vi "07Foot.vi"() -> ()   [LabVIEW 2020]
uses:
  <resource>/objmgr/daqmx.rc
  <vilib>/DAQmx/configure/timing.llb/DAQmx Timing (Sample Clock).vi
  <vilib>/Utility/file.llb/Read Delimited Spreadsheet (DBL).vi
  <vilib>/DAQmx/create/channels.llb/DAQmx Create Channel (DI-Digital Input).vi
  <vilib>/Utility/file.llb/Write Delimited Spreadsheet (DBL).vi
  <vilib>/Instr/_visa.llb/VISA Configure Serial Port (Serial Instr).vi
  07FootGlobals.vi
panel:
  in  "Tab Control":enum32{"Page 1", "Page 2"}(tab)
  out "NEXT DURATION":dbl format="%#.1f"
  out "NEXT MPH":dbl min=0.0 max=12.0 step=0.1 format="%.1f"
  out "Time Left":dbl format="%#.0f"
  out "ESTOP":bool
  in  "ESTOP RESUME":bool
  out "MPH":dbl min=0.0 max=12.0 step=0.1 format="%.1f"
  out "ESTOP2":bool
  out "Report Location":path
  in  "TestScript":path=path "C:/LabVIEW VIs/TRMConsole/FootTime.txt"
  out "Waveform Graph":dbl[](graph)
  out "speed":dbl[](array[numeric])
  out "time":dbl[](array[numeric])
  out "dwell":dbl[](array[numeric])
  out "step":i32
  out "arraysize":i32
  out "x-y":u32
  out "appended path":path
  out "stopping":bool
  out "String":string
  in  "stop":bool
  out "MPH READ":u8
  in  "Serial Port":refnum<visa-resource-name>="COM8"
  in  "lines":tag="DAQMod1/port0"
  out "Enum":T1(ring)
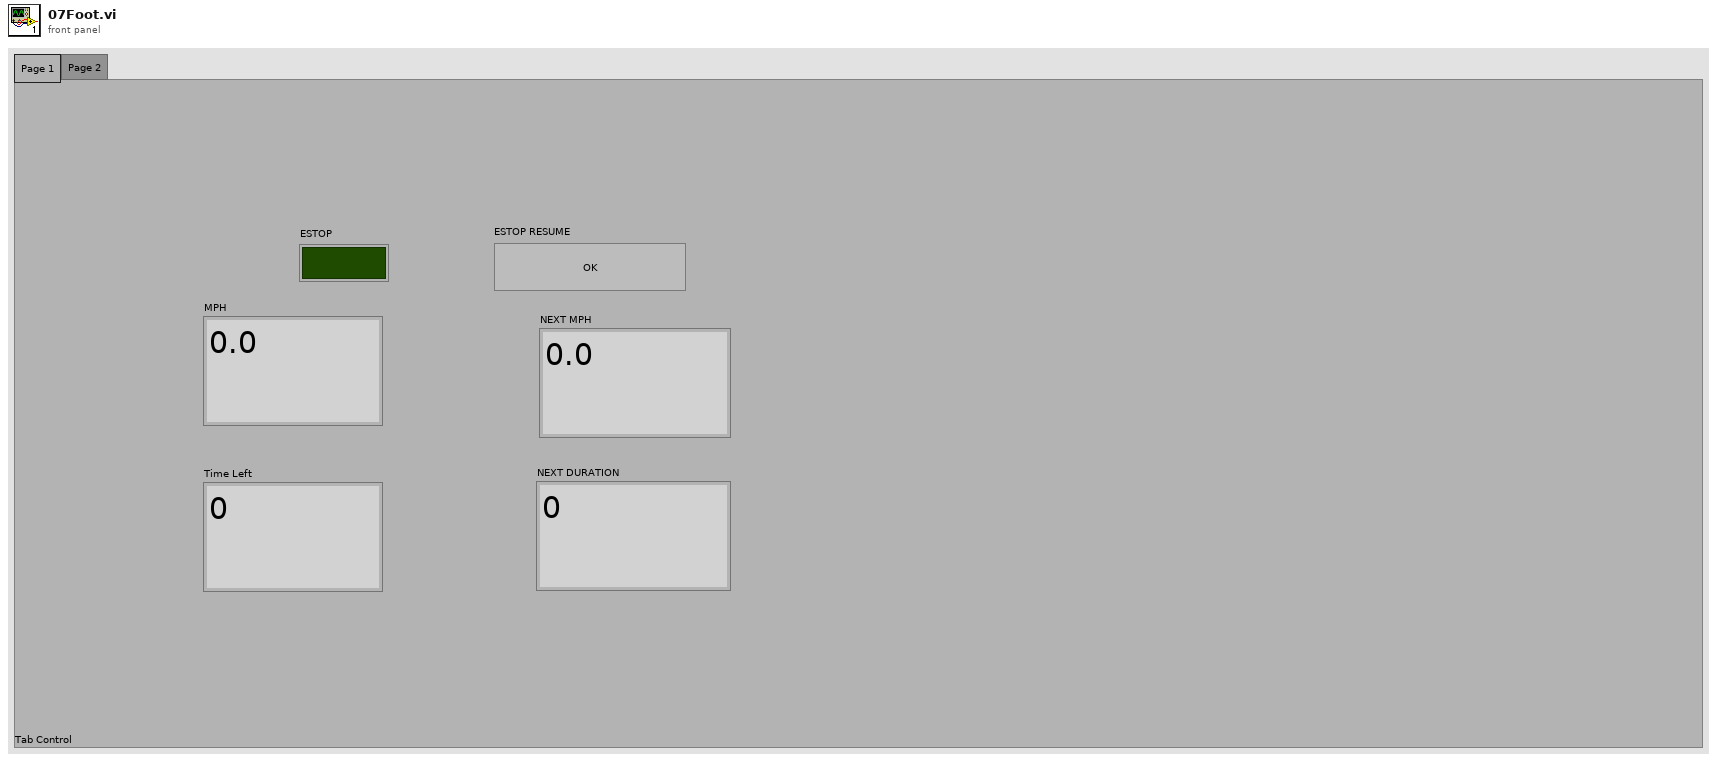
[diagram p1: front panel]
types:
  T1 = enum16{"Initialize", "SetMPH", "GetData", "CheckTiming", "CompressWave", "StartDAQ", "StopDAQ", "Dwell", "WaitforMPH", "ESTOP Wait", "ESTOP Resume"}
  T2 = enum16{"Initialize", "SetMPH", "GetData", "CheckTiming", "CompressWave", "StartDAQ", "StopDAQ", "Dwell", "WaitforMPH"}
  T3 = enum16{"Initialize", "SetMPH", "GetData", "CheckTiming", "CompressWave", "StartDAQ"}
  T4 = enum16{"Initialize", "SetMPH", "GetData", "CheckTiming", "CompressWave"}
  T5 = enum16{"Initialize", "SetMPH", "GetData", "CheckTiming", "CompressWave", "StartDAQ", "StopDAQ"}
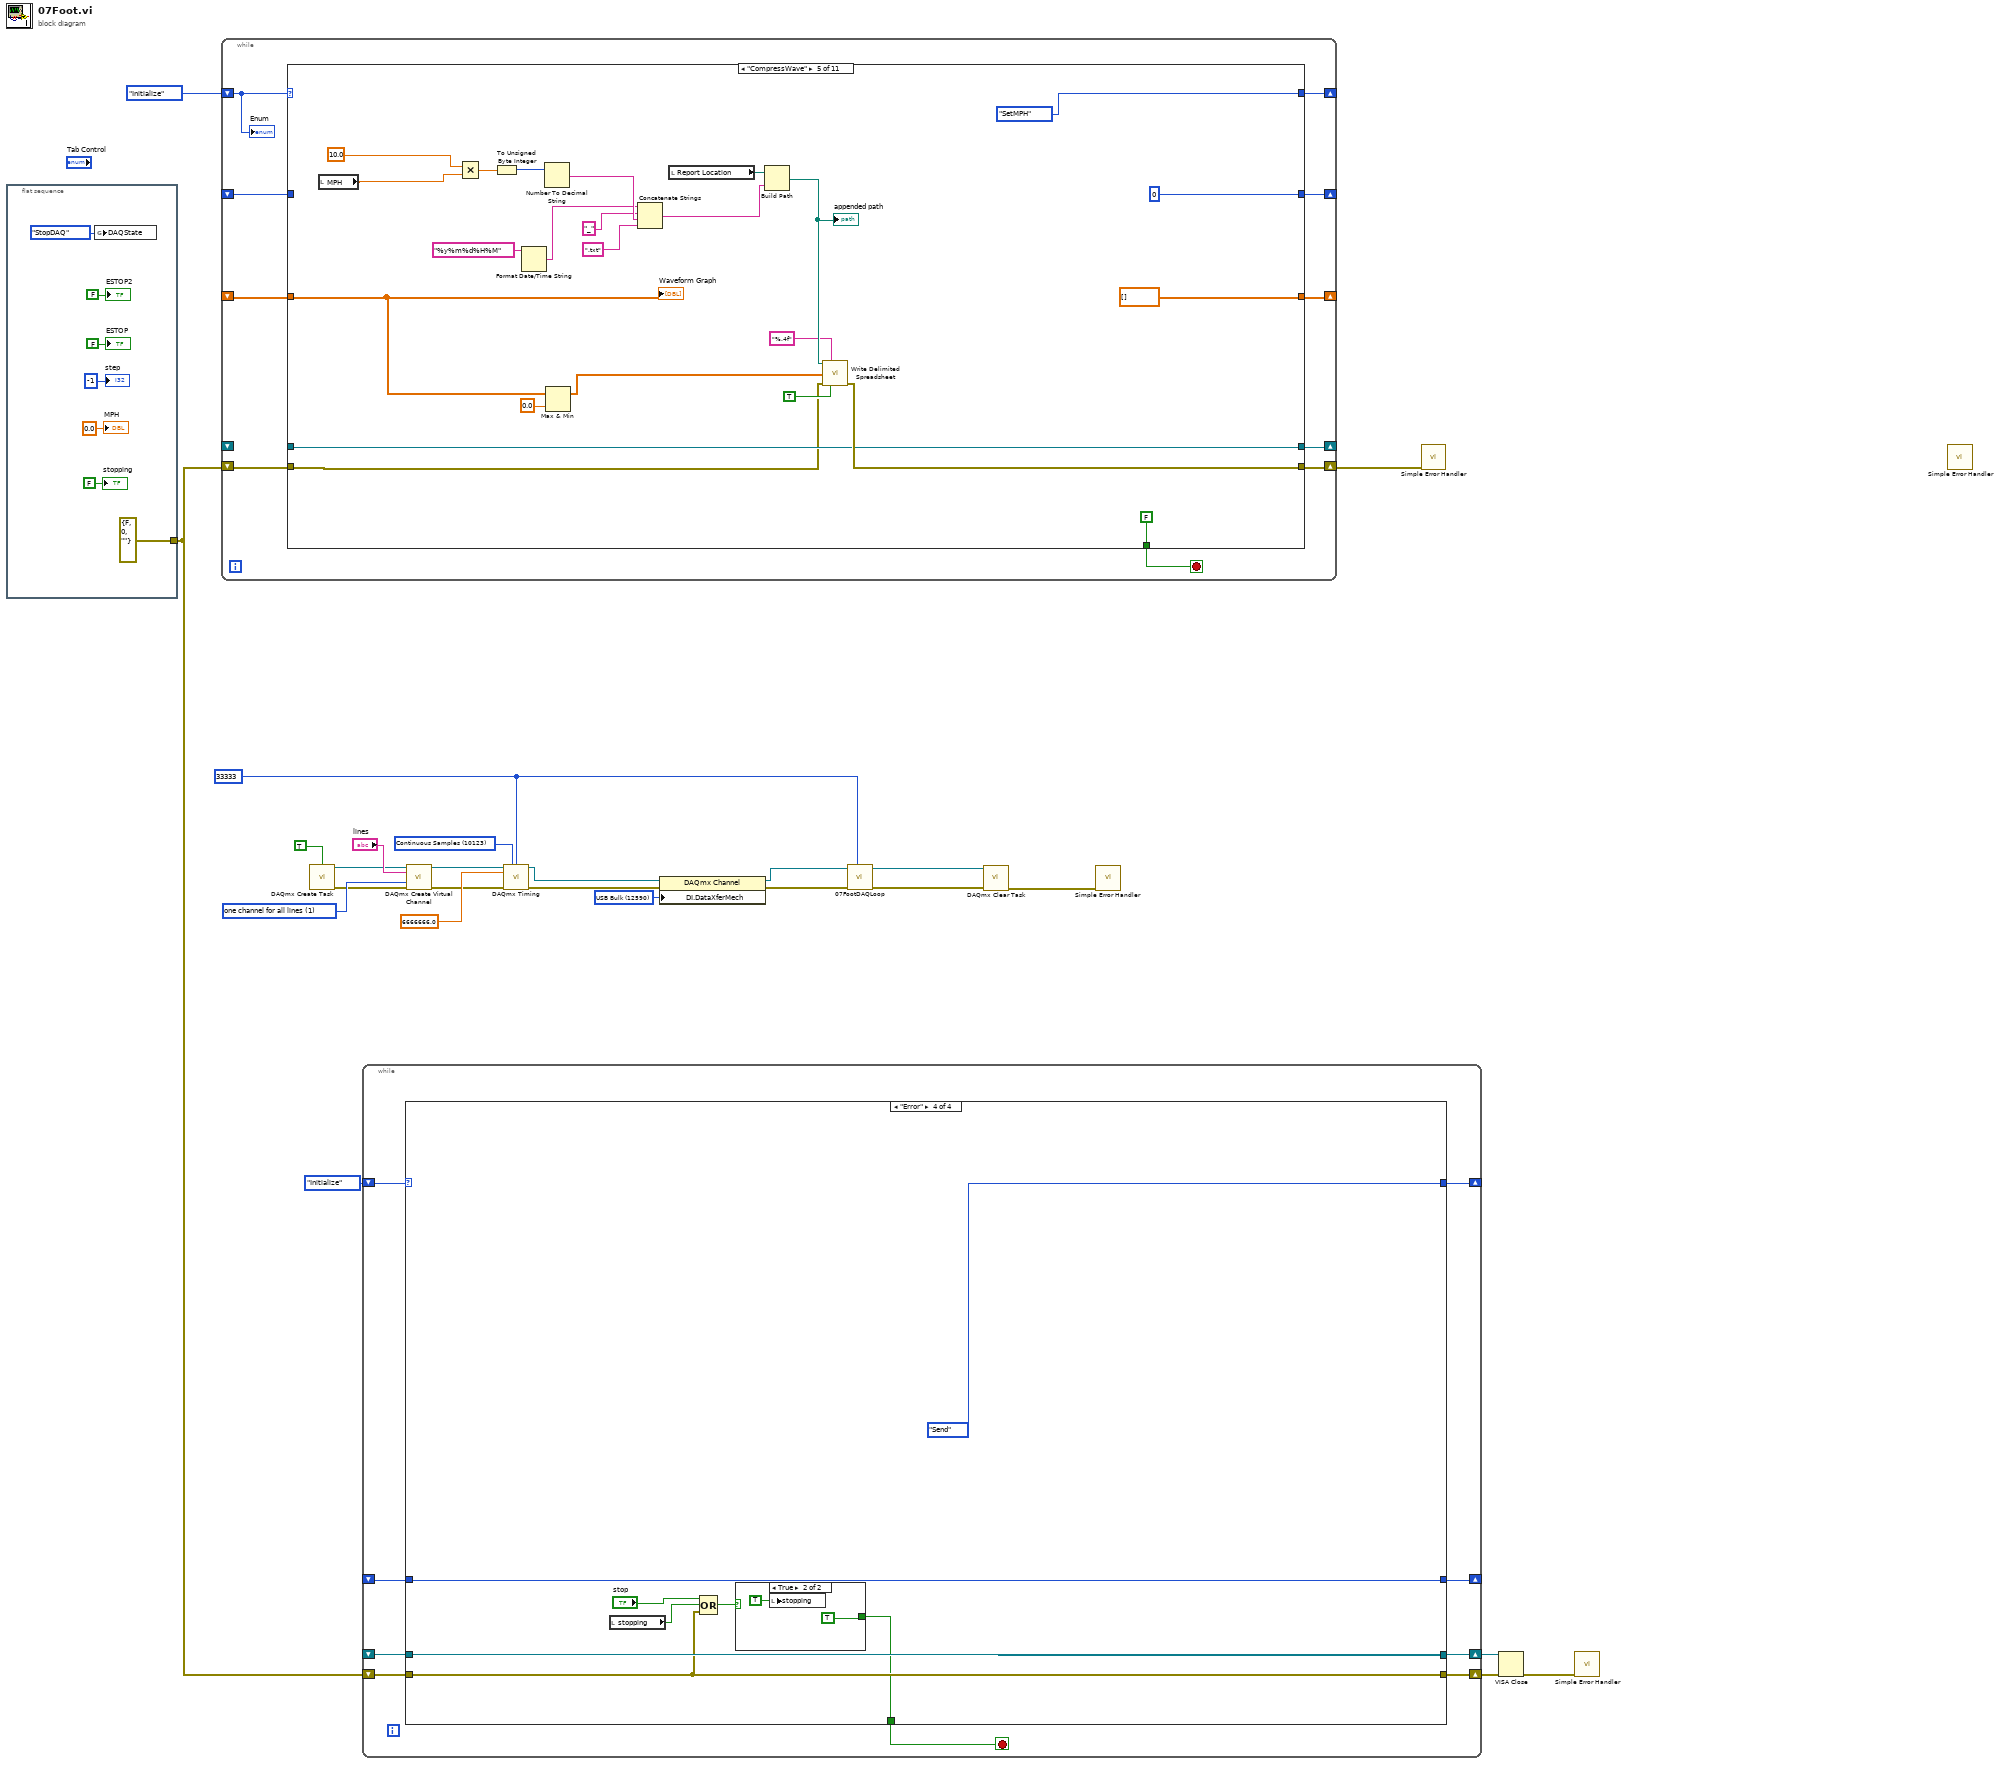
[diagram p0: block diagram]
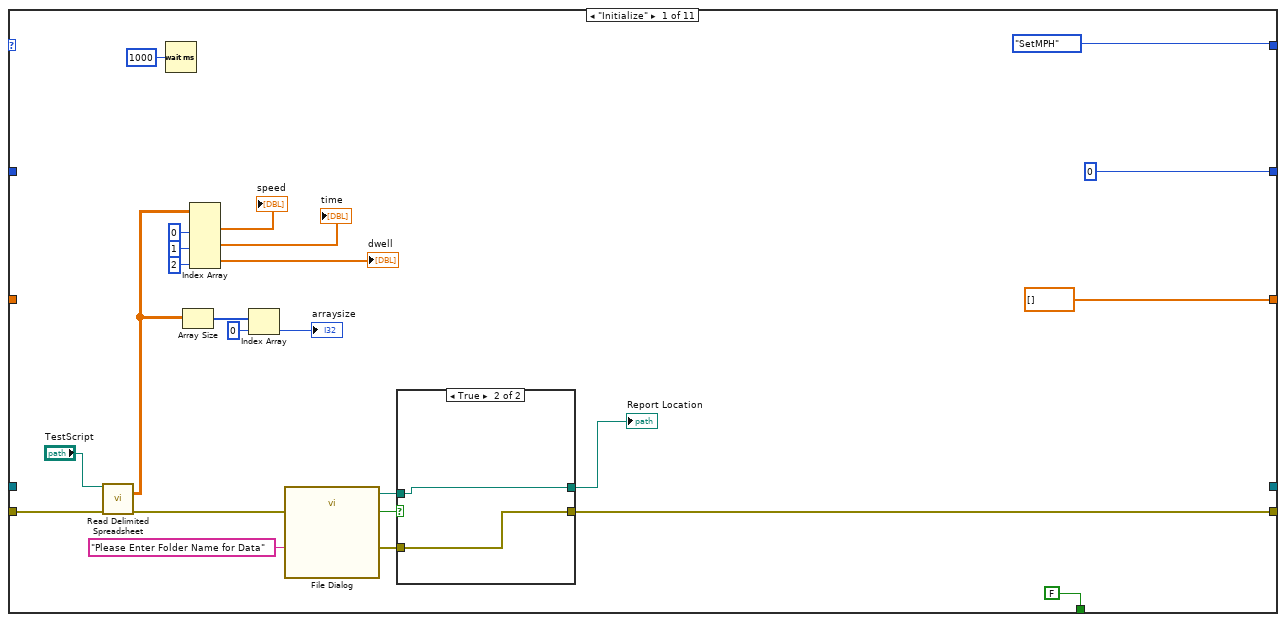
[diagram p2: hidden frame]
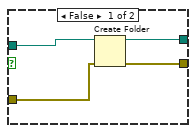
[diagram p3: hidden frame]
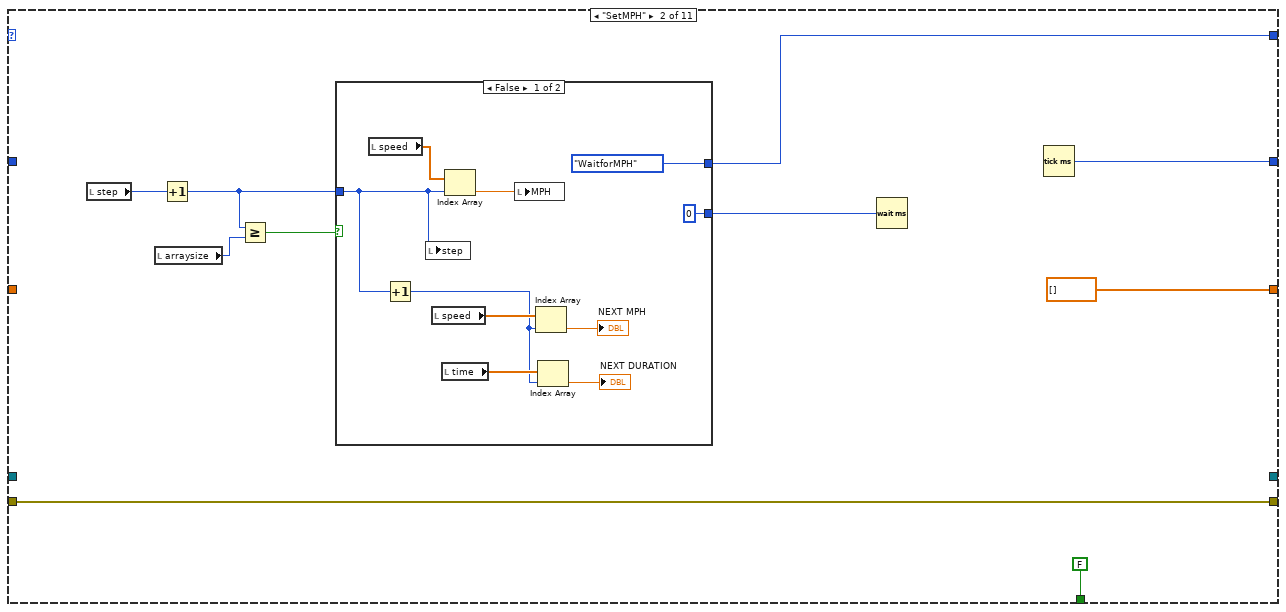
[diagram p4: hidden frame]
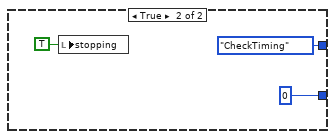
[diagram p5: hidden frame]
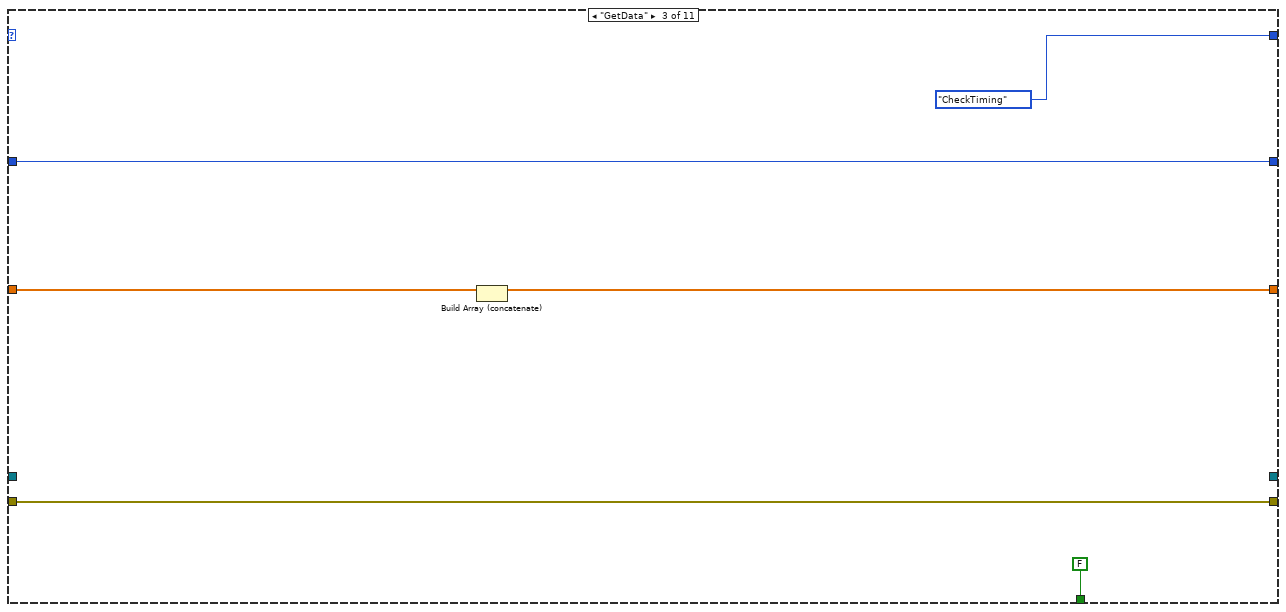
[diagram p6: hidden frame]
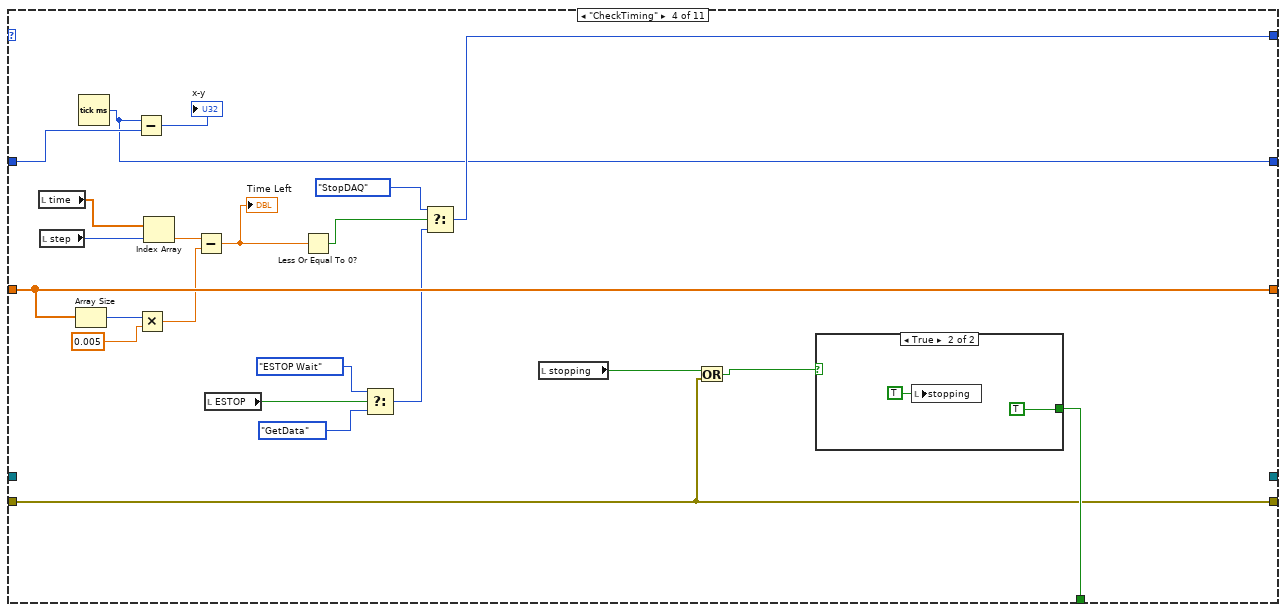
[diagram p7: hidden frame]
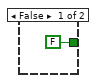
[diagram p8: hidden frame]
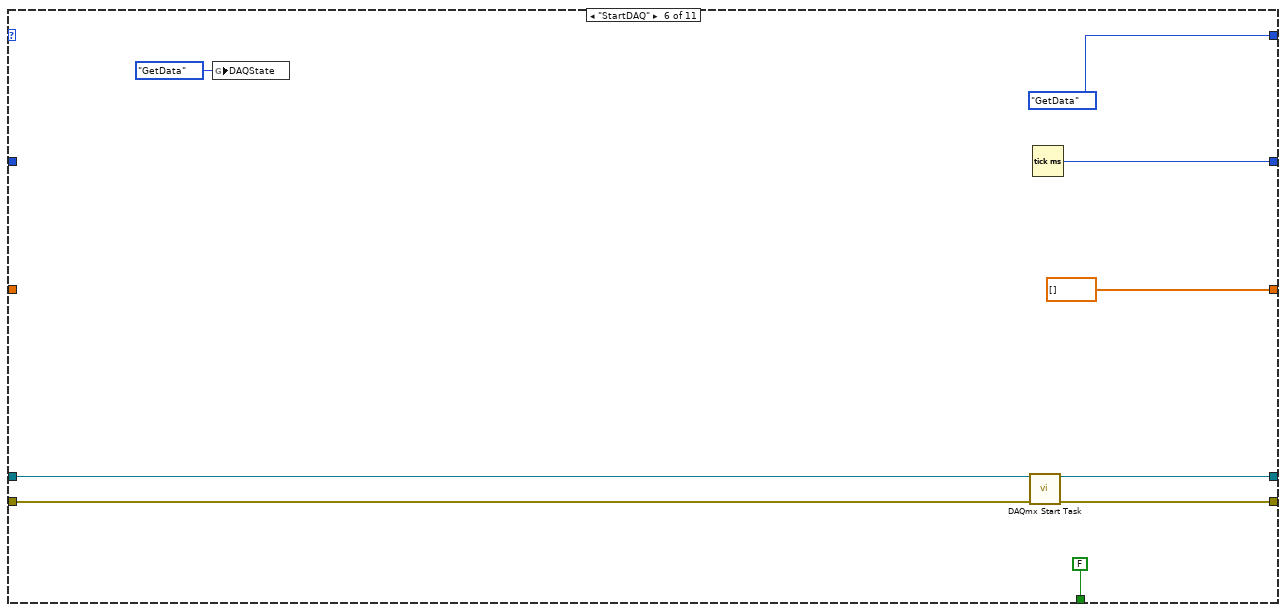
[diagram p9: hidden frame]
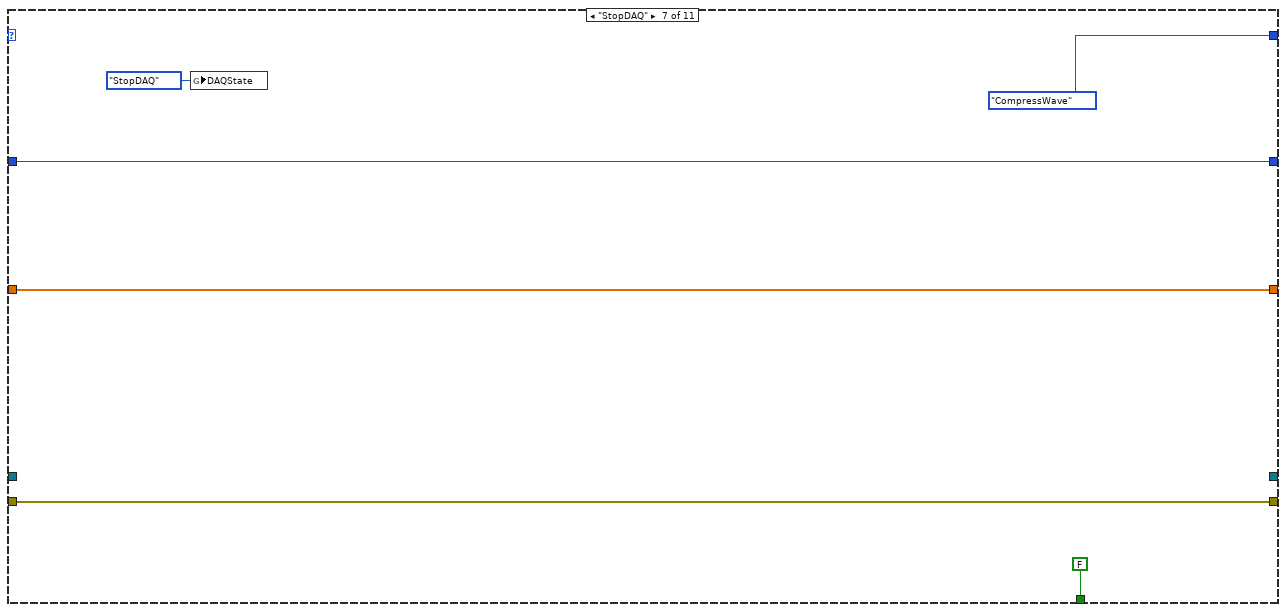
[diagram p10: hidden frame]
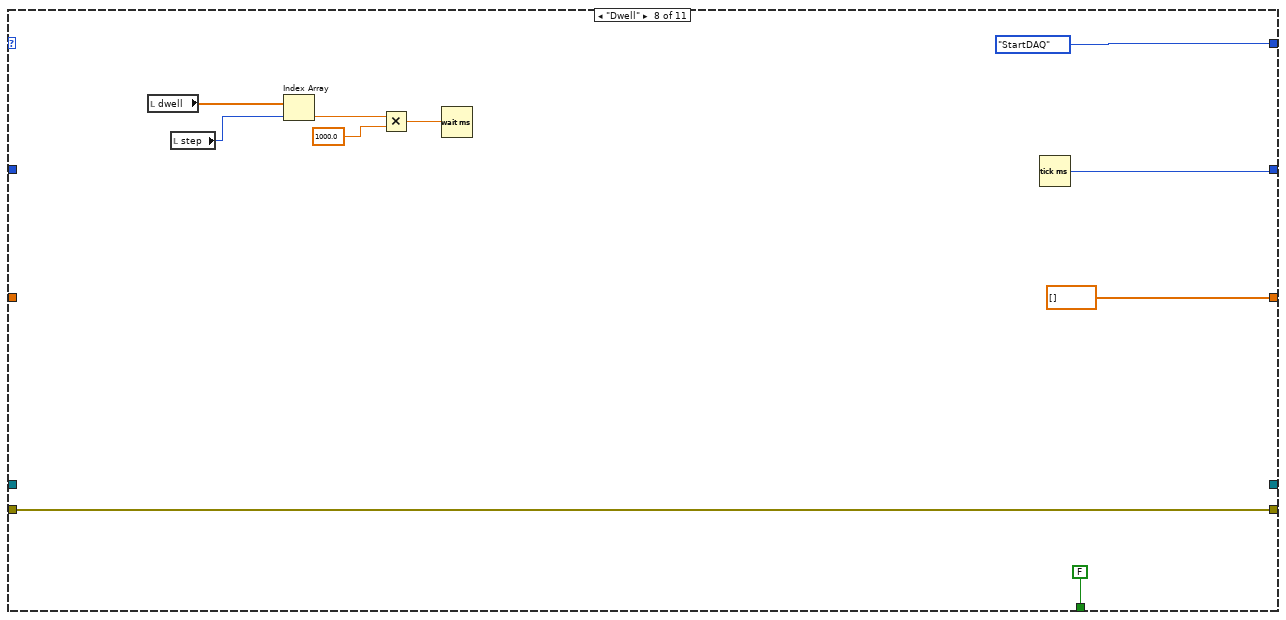
[diagram p11: hidden frame]
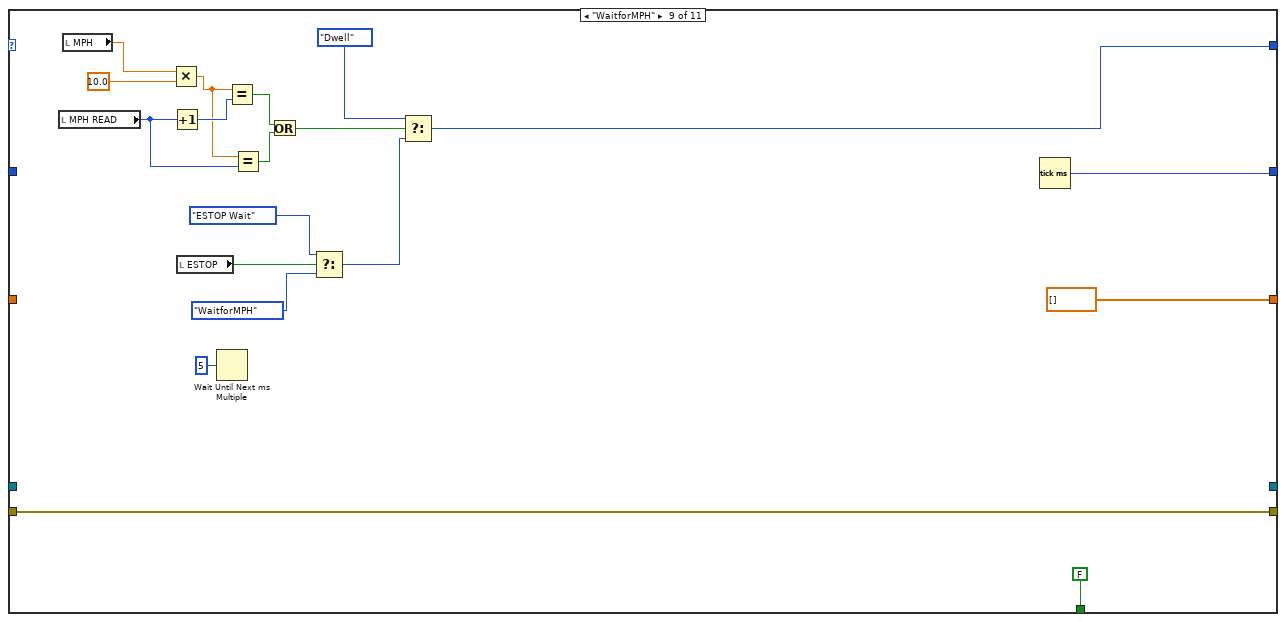
[diagram p12: hidden frame]
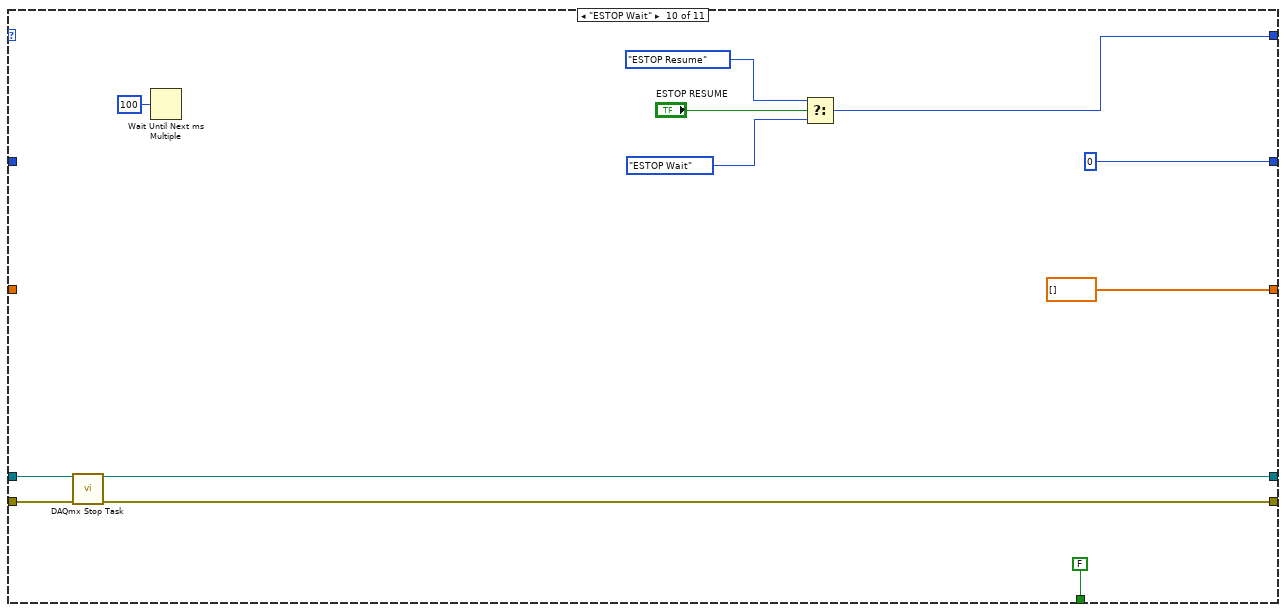
[diagram p13: hidden frame]
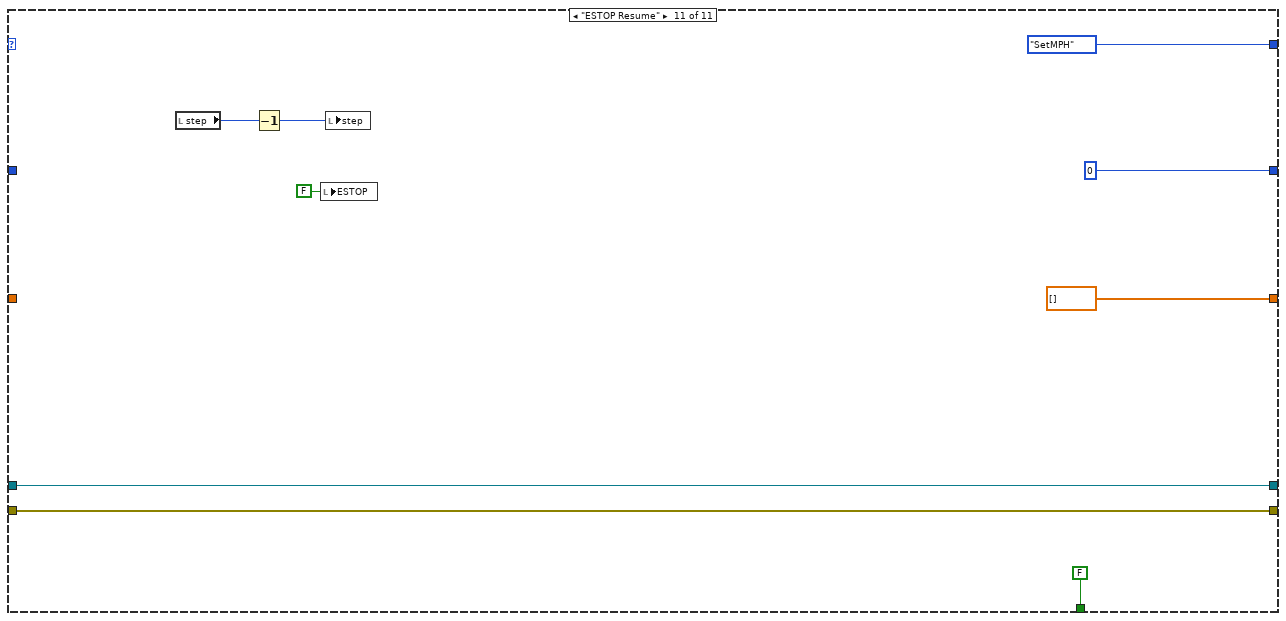
[diagram p14: hidden frame]
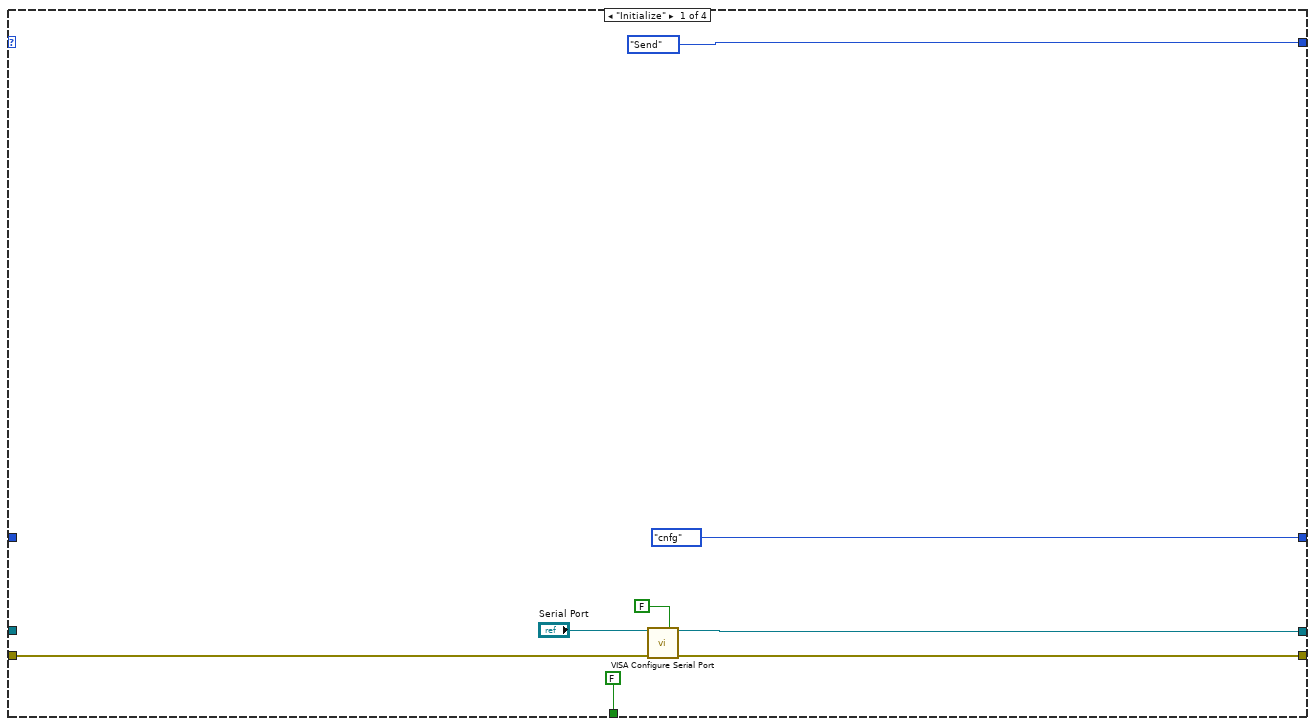
[diagram p15: hidden frame]
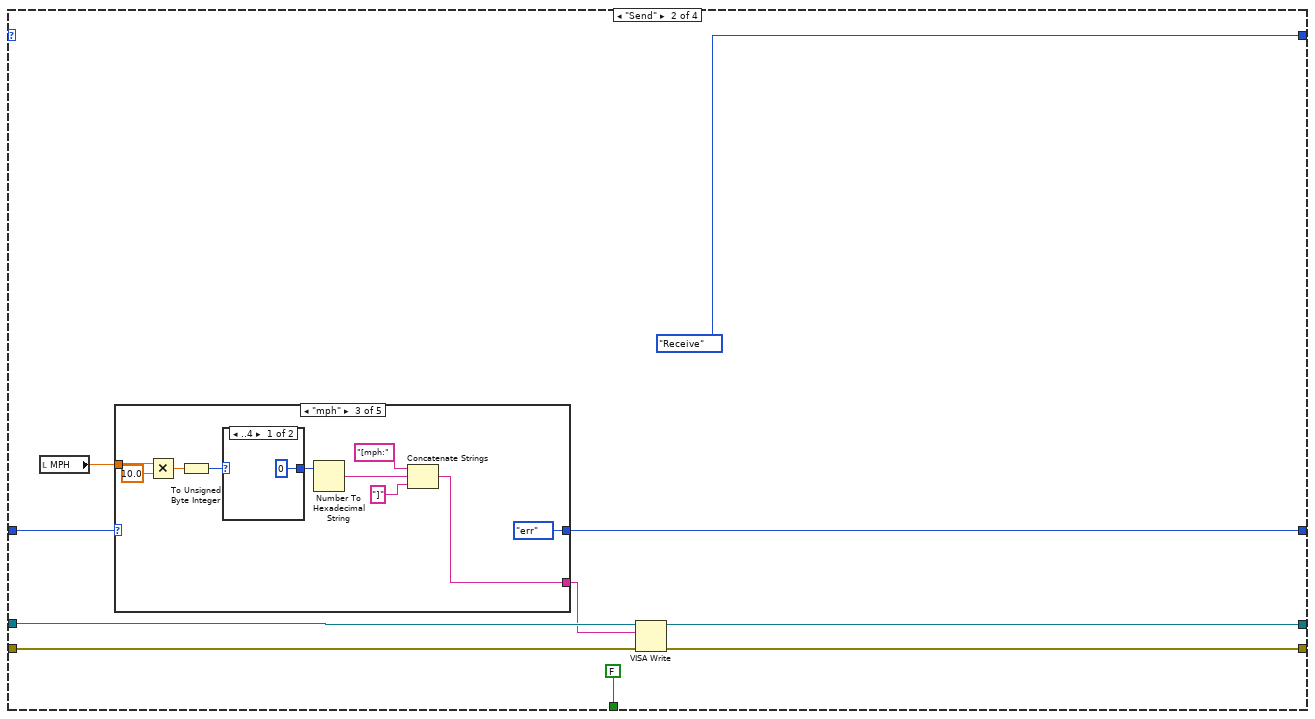
[diagram p16: hidden frame]
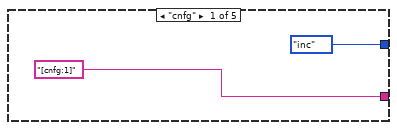
[diagram p17: hidden frame]
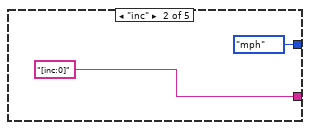
[diagram p18: hidden frame]
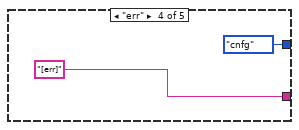
[diagram p20: hidden frame]
diagram:
  w19 = 12590 items=["DMA"=10054, "Interrupts"=10204, "Programmed I/O"=10264, "USB Bulk"=12590] ("DI.DataXferMech")
  w15 = 10123 items=["Finite Samples"=10178, "Continuous Samples"=10123, "Hardware Timed Single Point"=12522] ("sample mode")
  w10 = 1 items=["one channel for each line", "one channel for all lines"] ("line grouping")
  w5 = 33333 ("samples per channel")
  n1 = flat-sequence {
    tunnel: [errorcluster {"status"=FALSE, "code"=0, "source"=""} ("error constant")] -> w20
    frame #0 {
      n2 = global write "07FootGlobals.vi" "DAQState"(enum16{"GetData", "StopDAQ"}."StopDAQ" ("DAQState")) -> ()
      "stopping" <- FALSE ("stopping")
      "MPH" <- 0.0 ("MPH")
      "step" <- -1 ("step")
      "ESTOP" <- FALSE ("ESTOP")
      "ESTOP2" <- FALSE ("ESTOP2")
    }
  }
  n3 = while {
    shift-right: [w42] -> _
    shift-left: T1."Initialize" -> [w33]
    shift-right: [w40] -> _
    shift-left: _ -> [_]
    shift-right: [w39] -> w1
    shift-left: w20 -> [w38]
    shift-right: [w37] -> _
    shift-left: _ -> [w36]
    shift-right: [w35] -> _
    shift-left: _ -> [w34]
    stop <- w41 stop-if-true
    n4 = case shown="\"CompressWave\"" w33 {
      tunnel: [T1."SetMPH" w77 T4."CheckTiming" w117 T1."SetMPH" T3."GetData" T5."CompressWave" T2."StartDAQ" w187 w201 T1."SetMPH" ("f")] -> w42
      tunnel: [FALSE FALSE FALSE w122 FALSE FALSE FALSE FALSE FALSE FALSE FALSE] -> w41
      tunnel: [_ _ _ _ w134 w154 _ _ _ w196 w209] -> w40
      tunnel: [w43 w79 w96 w118 w147 w155 w161 w173 w192 w195 w210] -> w39
      tunnel: _ -> [_ _ _ _ w134 w153 _ _ _ w198 w209]
      tunnel: w38 -> [w62 w79 w96 w118 w133 w152 w161 w173 w192 w197 w210]
      tunnel: [u32 0 w78 w100 w102 u32 0 w158 w162 w175 w194 u32 0 ("millisecond timer value") u32 0 ("millisecond timer value")] -> w37
      tunnel: w36 -> [_ _ w100 w121 _ _ w162 _ _ _ _]
      tunnel: [dbl[] [] dbl[] [] w99 w116 dbl[] [] dbl[] [] w164 dbl[] [] dbl[] [] dbl[] [] dbl[] []] -> w35
      tunnel: w34 -> [_ _ w98 w116 w128 _ w164 _ _ _ _]
      frame "Initialize" {
        n5 = call-poly <vilib>:"Read Delimited Spreadsheet.vi"("file path (dialog if empty)"="TestScript", "error in (no error)"=w62) -> ("all rows"=w52:dbl[][], "error out"=w50:errorcluster)  [unwired: 8 in, 4 out]
        n6 = Wait (ms)(milliseconds to wait=u32 1000) -> ()  [unwired: 1 out]
        n7 = Array Size(array=w52) -> (size(s)=w55:i32[])
        n8 = Index Array(array=w52, index (col) #1=0 ("disabled index (col)"), index (col) #2=1 ("index (col)"), index (col) #3=2 ("index (col)")) -> (element #1=→"speed":dbl[], element #2=→"time":dbl[], element #3=→"dwell":dbl[])  [unwired: 3 in]
        n9 = Index Array(array=w55, index=0) -> (element=→"arraysize":i32)
        n10 = call "File Dialog"("prompt"="Please Enter Folder Name for Data", "error in"=w50) -> ("selected path"=w46:path, "exists"=w48:bool, "error out"=w47:errorcluster)  [unwired: 10 in, 1 out]
        n11 = case shown="True" w48 {
          tunnel: w47 -> [w70 w71]
          tunnel: w46 -> [w69 w72]
          tunnel: [w68 w71] -> w43
          tunnel: [w67 w72] -> w45
          frame False {
            n12 = Create Folder(path (use dialog)=w69, error in=w70) -> (created path=w67:path, error out=w68:errorcluster)  [unwired: 1 in, 1 out]
          }
          frame True {
          }
        }
        "Report Location" <- w45
      }
      frame "SetMPH" {
        n13 = local read "step"() -> (w74:i32)
        n14 = local read "arraysize"() -> (w76:i32)
        n15 = Increment(x=w74) -> (x+1=w73:i32)
        n16 = Greater Or Equal?(x=w73, y=w76) -> (x >= y?=w75:bool)
        n17 = case shown="False" w75 {
          tunnel: [u32 0 ("milliseconds to wait") u32 0 ("milliseconds to wait")] -> w81
          tunnel: [T2."WaitforMPH" T3."CheckTiming"] -> w77
          tunnel: w73 -> [w88 _]
          frame False {
            n18 = local read "speed"() -> (w91:dbl[])
            n19 = Increment(x=w88) -> (x+1=w83:i32)
            n20 = local write "step"(w88) -> ()
            n21 = local read "speed"() -> (w87:dbl[])
            n22 = local read "time"() -> (w84:dbl[])
            n23 = Index Array(array=w91, index=w88) -> (element=w90:dbl)
            n24 = local write "MPH"(w90) -> ()
            n25 = Index Array(array=w87, index=w83) -> (element=→"NEXT MPH":dbl)
            n26 = Index Array(array=w84, index=w83) -> (element=→"NEXT DURATION":dbl)
          }
          frame True {
            n27 = local write "stopping"(TRUE ("stopping")) -> ()
          }
        }
        n28 = Wait (ms)(milliseconds to wait=w81) -> ()  [unwired: 1 out]
        n29 = Tick Count (ms)() -> (millisecond timer value=w78:u32)
      }
      frame "GetData" {
        n30 = Build Array (concatenate)(w98) -> (w99:dbl[])  [unwired: 1 in]
      }
      frame "CheckTiming" {
        n31 = local read "time"() -> (w113:dbl[])
        n32 = local read "step"() -> (w112:i32)
        n33 = Array Size(array=w116) -> (size(s)=w115:i32)
        n34 = Tick Count (ms)() -> (millisecond timer value=w102:u32)
        n35 = Subtract(x=w102, y=w121) -> (x-y=→"x-y":u32)
        n36 = Multiply(x=w115, y=0.005) -> (x*y=w105:dbl)
        n37 = Index Array(array=w113, index=w112) -> (element=w106:dbl)
        n38 = Subtract(x=w106, y=w105) -> (x-y=w104:dbl)
        "Time Left" <- w104
        n39 = local read "ESTOP"() -> (w109:bool)
        n40 = Less Or Equal To 0?(x=w104) -> (x <= 0?=w103:bool)
        n41 = Select(t=T1."ESTOP Wait", s=w109, f=T1."GetData") -> (s? t:f=w107:T1)
        n42 = Select(t=T1."StopDAQ", s=w103, f=w107) -> (s? t:f=w117:T1)
        n43 = local read "stopping"() -> (w120:bool)
        n44 = Or(x=w120, y=w118) -> (x .or. y?=w119:bool)
        n45 = case shown="True" w119 {
          tunnel: [FALSE TRUE] -> w122
          frame False {
          }
          frame True {
            n46 = local write "stopping"(TRUE ("stopping")) -> ()
          }
        }
      }
      frame "CompressWave" {
        n47 = local read "MPH"() -> (w137:dbl)
        n48 = Multiply(x=10.0, y=w137) -> (x*y=w140:dbl)
        n49 = To Unsigned Byte Integer(number=w140) -> (unsigned 8bit integer=w139:u8)
        n50 = Format Date/Time String(time format string (%c)="%y%m%d%H%M") -> (date/time string=w129:string)  [unwired: 2 in]
        n51 = Number To Decimal String(number=w139) -> (decimal integer string=w138:string)  [unwired: 1 in]
        n52 = Max & Min(x=w128, y=0.0) -> (max(x,y)=w135:dbl[])  [unwired: 1 out]
        n53 = Concatenate Strings(w129, "_" ("string"), w138, ".txt" ("string")) -> (w143:string)
        n54 = local read "Report Location"() -> (w132:path)
        n55 = Build Path(base path=w132, name or relative path=w143) -> (appended path=w142:path)
        "appended path" <- w142
        n56 = call-poly <vilib>:"Write Delimited Spreadsheet.vi"("file path (dialog if empty)"=w142, "format (%.3f)"="%.4f", "1D data"=w135, "error in (no error)"=w133, "transpose? (no:F)"=TRUE ("transpose? (F)")) -> ("error out"=w147:errorcluster)  [unwired: 9 in, 1 out]
        "Waveform Graph" <- w128
      }
      frame "StartDAQ" {
        n57 = global write "07FootGlobals.vi" "DAQState"(enum16{"GetData", "StopDAQ", "Quit"}."GetData" ("DAQState")) -> ()
        n58 = call <vilib>:"DAQmx Start Task.vi"("task/channels in"=w153, "error in"=w152) -> ("task out"=w154:refnum<k21>, "error out"=w155:errorcluster)  [unwired: 12 in]
        n59 = Tick Count (ms)() -> (millisecond timer value=w158:u32)
      }
      frame "StopDAQ" {
        n60 = global write "07FootGlobals.vi" "DAQState"(enum16{"GetData", "StopDAQ", "Quit"}."StopDAQ" ("DAQState")) -> ()
      }
      frame "Dwell" {
        n61 = local read "dwell"() -> (w171:dbl[])
        n62 = local read "step"() -> (w170:i32)
        n63 = Index Array(array=w171, index=w170) -> (element=w169:dbl)
        n64 = Multiply(x=w169, y=1000.0) -> (x*y=w167:dbl)
        n65 = Wait (ms)(milliseconds to wait=w167) -> ()  [unwired: 1 out]
        n66 = Tick Count (ms)() -> (millisecond timer value=w175:u32)
      }
      frame "WaitforMPH" {
        n67 = local read "MPH READ"() -> (w179:u8)
        n68 = local read "MPH"() -> (w190:dbl)
        n69 = Multiply(x=w190, y=10.0) -> (x*y=w180:dbl)
        n70 = Increment(x=w179) -> (x+1=w188:u8)
        n71 = local read "ESTOP"() -> (w185:bool)
        n72 = Wait Until Next ms Multiple(millisecond multiple=u32 5) -> ()  [unwired: 1 out]
        n73 = Equal?(x=w180, y=w188) -> (x = y?=w177:bool)
        n74 = Equal?(x=w180, y=w179) -> (x = y?=w178:bool)
        n75 = Or(x=w177, y=w178) -> (x .or. y?=w176:bool)
        n76 = Select(t=T1."ESTOP Wait", s=w185, f=T1."WaitforMPH") -> (s? t:f=w182:T1)
        n77 = Select(t=T1."Dwell", s=w176, f=w182) -> (s? t:f=w187:T1)
        n78 = Tick Count (ms)() -> (millisecond timer value=w194:u32)
      }
      frame "ESTOP Wait" {
        n79 = call <vilib>:"DAQmx Stop Task.vi"("task/channels in"=w198, "error in"=w197) -> ("task out"=w196:refnum<k21>, "error out"=w195:errorcluster)  [unwired: 12 in]
        n80 = Wait Until Next ms Multiple(millisecond multiple=u32 100) -> ()  [unwired: 1 out]
        n81 = Select(t=T1."ESTOP Resume", s="ESTOP RESUME", f=T1."ESTOP Wait") -> (s? t:f=w201:T1)
      }
      frame "ESTOP Resume" {
        n82 = local read "step"() -> (w215:i32)
        n83 = Decrement(x=w215) -> (x-1=w214:i32)
        n84 = local write "ESTOP"(FALSE ("ESTOP")) -> ()
        n85 = local write "step"(w214) -> ()
      }
    }
    "Enum" <- w33
  }
  n86 = call <vilib>:"DAQmx Create Task.vi"("auto cleanup"=TRUE) -> ("task out"=w8:refnum<k21>, "error out"=w9:errorcluster)  [unwired: 13 in]
  n87 = while {
    shift-right: [w220] -> w23
    shift-left: w20 -> [w224]
    shift-right: [w221] -> w24
    shift-left: _ -> [w223]
    shift-right: [w219] -> _
    shift-left: enum16{"Initialize", "Send", "Receive", "Error"}."Initialize" -> [w222]
    shift-right: [w218] -> _
    shift-left: _ -> [w217]
    stop <- w216 stop-if-true
    n88 = case shown="\"Error\"" w222 {
      tunnel: w224 -> [w228 w240 w279 w299]
      tunnel: w223 -> [_ w239 w278 w303]
      tunnel: [w230 w242 w277 w303] -> w221
      tunnel: [w229 w241 w271 w299] -> w220
      tunnel: [enum16{"Initialize", "Send", "Receive", "Error"}."Send" enum16{"Initialize", "Send", "Receive", "Error"}."Receive" enum16{"Initialize", "Send", "Receive", "Error"}."Error" enum16{"Initialize", "Send", "Receive", "Error"}."Send"] -> w219
      tunnel: [enum16{"cnfg", "inc", "mph", "err", "RSET"}."cnfg" w236 w265 w304] -> w218
      tunnel: w217 -> [_ w237 w272 w304]
      tunnel: [FALSE FALSE FALSE w298] -> w216
      frame "Initialize" {
        n89 = call-poly "VISA Configure Serial Port"("VISA resource name"="Serial Port", "Enable Termination\nChar (T)"=FALSE ("Enable Termination\nChar (T)"), "error in (no error)"=w228) -> ("VISA resource name out"=w230:refnum<visa-resource-name>, "error out"=w229:errorcluster)  [unwired: 11 in]
      }
      frame "Send" {
        n90 = local read "MPH"() -> (w233:dbl)
        n91 = case shown="\"mph\"" w237 {
          tunnel: ["[cnfg:1]" "[inc:0]" w247 "[err]" "[RSET]"] -> w238
          tunnel: w233 -> [_ _ w256 _ _]
          tunnel: [enum16{"cnfg", "inc", "mph", "err", "RSET"}."inc" enum16{"cnfg", "inc", "mph", "err", "RSET"}."mph" enum16{"cnfg", "inc", "mph", "err", "RSET"}."err" enum16{"cnfg", "inc", "mph", "err", "RSET"}."cnfg" enum16{"cnfg", "inc", "mph", "err", "RSET"}."cnfg"] -> w236
          frame "cnfg" {
          }
          frame "inc" {
          }
          frame "mph" {
            n92 = Multiply(x=w256, y=10.0) -> (x*y=w250:dbl)
            n93 = To Unsigned Byte Integer(number=w250) -> (unsigned 8bit integer=w249:u8)
            n94 = case shown="..4" w249 {
              selector: w249 -> [_ w258]
              tunnel: [u8 0 w258] -> w248
              frame ..4 {
              }
              frame 5.. {
              }
            }
            n95 = Number To Hexadecimal String(2:w248) -> (0:w253:string)  [unwired: 1 in]
            n96 = Concatenate Strings("[mph:" ("string"), w253, "]" ("string")) -> (w247:string)
          }
          frame "err" {
          }
          frame "RSET" {
          }
        }
        n97 = VISA Write(VISA resource name=w239, write buffer=w238, error in (no error)=w240) -> (VISA resource name out=w242:refnum<visa-resource-name>, error out=w241:errorcluster)  [unwired: 1 out]
      }
      frame "Receive" {
        n98 = flat-sequence {
          tunnel: w278 -> [w296]
          tunnel: [w296] -> w283
          frame #0 {
            n99 = Wait Until Next ms Multiple(millisecond multiple=u32 250) -> ()  [unwired: 1 out]
          }
        }
        n100 = property class="Serial Instr"(reference=w283, error in=w279) -> (reference out=w281:refnum<visa-resource-name>, error out=w282:errorcluster, "Bytes at Port"=w280:u32)
        n101 = VISA Read(VISA resource name=w281, byte count=w280, error in (no error)=w282) -> (VISA resource name out=w277:refnum<visa-resource-name>, read buffer=w266:string, error out=w271:errorcluster)  [unwired: 1 out]
        n102 = Match Pattern(string=w266, regular expression="\\[mph:") -> (after substring=w268:string, offset past match=w269:i32)  [unwired: 1 in, 2 out]
        n103 = Match Pattern(string=w266, regular expression="\\[err:") -> (offset past match=w273:i32)  [unwired: 1 in, 3 out]
        n104 = case shown="Default" w269 {
          tunnel: w268 -> [w290 _]
          frame Default {
            n105 = Hexadecimal String To Number(string=w290, default (0uL)=u8 0 ("default (0 I32)")) -> (number=→"MPH READ":u8)  [unwired: 1 in, 1 out]
          }
          frame -1 {
          }
        }
        n106 = case shown="Default" w273 {
          tunnel: [enum16{"cnfg", "inc", "mph", "err", "RSET"}."RSET" w295] -> w267
          tunnel: w272 -> [_ w295]
          tunnel: w266 -> [w291 _]
          frame Default {
            (unwired) "%y%m%d%H%M" ("time format string (%c)")
            n107 = Format Date/Time String() -> (date/time string=w292:string)  [unwired: 3 in]
            n108 = Concatenate Strings(w292, w291) -> (→"String":string)
          }
          frame -1 {
          }
        }
        n109 = Match Pattern(string=w266, regular expression="\\[ESTOP:BAD\\]") -> (offset past match=w264:i32)  [unwired: 1 in, 3 out]
        n110 = case shown="Default" w264 {
          tunnel: w267 -> [_ w287]
          tunnel: [enum16{"cnfg", "inc", "mph", "err", "RSET"}."RSET" w287] -> w265
          frame Default {
            n111 = local write "ESTOP"(TRUE ("ESTOP")) -> ()
            n112 = local write "MPH"(0.0 ("MPH")) -> ()
          }
          frame -1 {
          }
        }
      }
      frame "Error" {
        n113 = local read "stopping"() -> (w300:bool)
        n114 = Compound Arithmetic op=OR("stop", w300, w299) -> (w302:bool)
        n115 = case shown="True" w302 {
          tunnel: [FALSE TRUE] -> w298
          frame False {
          }
          frame True {
            n116 = local write "stopping"(TRUE ("stopping")) -> ()
          }
        }
      }
    }
  }
  n117 = call-poly <vilib>:"DAQmx Create Virtual Channel.vi"("task in"=w8, "lines"="lines", "line grouping"=w10, "error in"=w9) -> ("task out"=w14:refnum<k21>, "error out"=w13:errorcluster)  [unwired: 10 in]
  n118 = call-poly <vilib>:"DAQmx Timing.vi"("task/channels in"=w14, "sample mode"=w15, "samples per channel"=w5, "rate"=6666666.0, "error in"=w13) -> ("task out"=w17:refnum<k21>, "error out"=w18:errorcluster)  [unwired: 9 in]
  n119 = property class="DAQmx Channel"(reference=w17, error in=w18, "DI.DataXferMech"=w19) -> (reference out=w6:refnum<k21>, error out=w7:errorcluster)
  n120 = call "07FootDAQLoop.vi"("samples per channel"=w5, "error in (no error)"=w7, "task in"=w6) -> ("error out"=w3:errorcluster, "task out"=w4:refnum<k21>)  [unwired: 7 in]
  n121 = call <vilib>:"DAQmx Clear Task.vi"("task in"=w4, "error in"=w3) -> ("error out"=w2:errorcluster)  [unwired: 13 in]
  n122 = call <vilib>:"Simple Error Handler.vi"("error in (no error)"=w2) -> ()  [unwired: 4 in, 5 out]
  n123 = call <vilib>:"Simple Error Handler.vi"("error in (no error)"=w1) -> ()  [unwired: 4 in, 5 out]
  n124 = VISA Close(VISA resource name=w24, error in (no error)=w23) -> (error out=w22:errorcluster)
  n125 = call <vilib>:"Simple Error Handler.vi"("error in (no error)"=w22) -> ()  [unwired: 4 in, 5 out]
  n126 = call <vilib>:"Simple Error Handler.vi"() -> ()  [unwired: 5 in, 5 out]
